vi "Pockels-Correct ref time for FPGA.vi"(9 "Fine tuning multiplier":dbl=1.5 format="%#_13g", 10 "Time for main img line OR for a single POI (ms)":dbl, 11 "Actual resulting time between ref triggers (ms)":dbl) -> (1 "Ref Scan Cycles":dbl, 3 "Adjusted time between ref \ntriggers sent to the FPGA (ms)":dbl)   [LabVIEW 2017]
panel:
  # "<--This is the time between reference frame triggers in FPGA clock cycles"
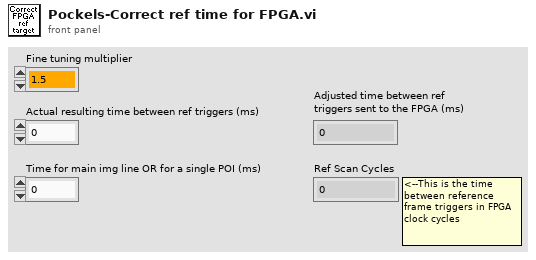
[diagram p1: front panel]
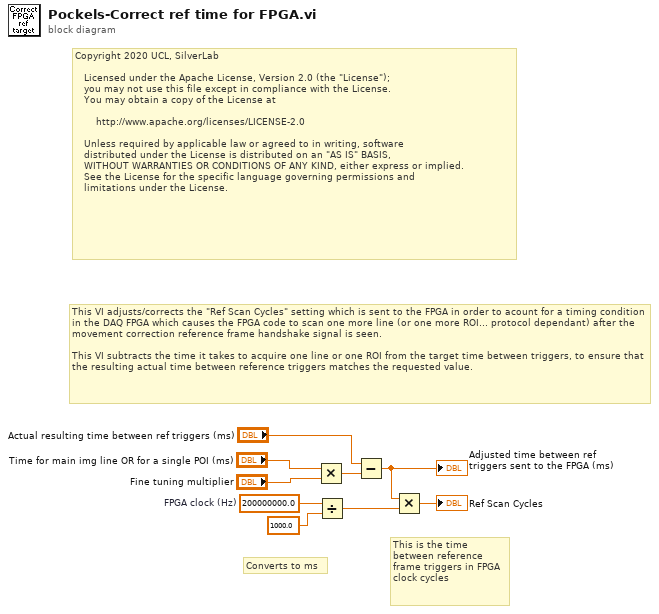
[diagram p0: block diagram]
diagram:
  w6 = 200000000.0  # FPGA clock (Hz)
  # "Copyright 2020 UCL, SilverLab\n \n   Licensed under the Apache License, Version 2.0 (the \"License\");\n   you may not use this file except in compliance with the License.\n   You may obtain a copy of the License at\n \n       http://www.apache.org/licenses/LICENSE-2.0\n \n   Unless required by applicable law or agreed to in writing, software\n   distributed under the License is distributed on an \"AS IS\" BASIS,\n   WITHOUT WARRANTIES OR CONDITIONS OF ANY KIND, either express or implied.\n   See the License for the specific language governing permissions and\n   limitations under the License."
  # "This is the time between reference frame triggers in FPGA clock cycles"
  # "This VI adjusts/corrects the \"Ref Scan Cycles\" setting which is sent to the FPGA in order to acount for a timing condition in the DAQ FPGA which causes the FPGA code to scan one more line (or one more ROI... protocol dependant) after the movement correction reference frame handshake signal is seen.\n\nThis VI subtracts the time it takes to acquire one line or one ROI from the target time between triggers, to ensure that the resulting actual time between reference triggers matches the requested value."
  # "Converts to ms"
  n1 = Multiply(x="Time for main img line OR for a single POI (ms)", y="Fine tuning multiplier") -> (x*y=w4:dbl)
  n2 = Divide(x=w6, y=1000.0) -> (x/y=w7:dbl)
  n3 = Subtract(x="Actual resulting time between ref triggers (ms)", y=w4) -> (x-y=w8:dbl)
  "Adjusted time between ref \ntriggers sent to the FPGA (ms)" <- w8
  n4 = Multiply(x=w8, y=w7) -> (x*y=→"Ref Scan Cycles":dbl)
